vi "ExitNowAllLoops.vi"(8 "error in (no error)":errorcluster, 11 "MessageQues":T1) -> (0 "error out":errorcluster)   [LabVIEW 2019]
doc: "Send ExitNow message to all loops.\n\n Execute all que operations even if there is an error in.\n\nBolder Software LLC"
uses:
  VXM Main Test App/MultipleMessageQues vxm.ctl
  MessageQue.ctl
  MessageCluster.ctl
  MessageQue.lvlib
panel:
  # "SaveData Ques\nDisplay Que\nDisplayNotifier"
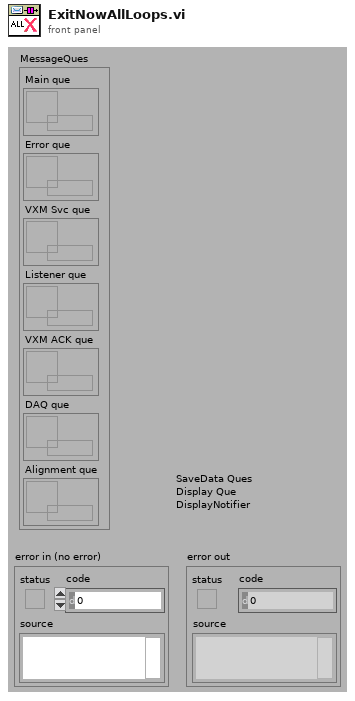
[diagram p1: front panel]
types:
  T1 = typedef "MultipleMessageQues vxm.ctl" = cluster{"Main que":T2, "Error que":T2, "VXM Svc que":T2, "Listener que":T2, "VXM ACK que":T2, "DAQ que":T2, "Alignment que":T2}
  T2 = typedef "MessageQue.lvlib/MessageQue.ctl" = refnum<queue>
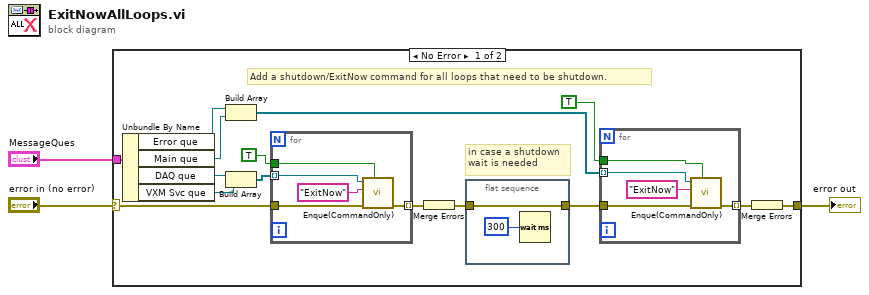
[diagram p0: block diagram]
diagram:
  n1 = case shown="No Error" "error in (no error)" {
    selector: "error in (no error)" -> [w18 w31]
    tunnel: [w11 w31] -> w2
    tunnel: "MessageQues" -> [w15 _]
    frame No Error {
      # "Add a shutdown/ExitNow command for all loops that need to be shutdown."
      # "in case a shutdown\nwait is needed"
      n2 = Unbundle By Name(w15) -> ("Error que"=w6:T2, "Main que"=w5:T2, "DAQ que"=w13:T2, "VXM Svc que"=w4:T2)
      n3 = Build Array(w6, w5) -> (w9:T2[])
      n4 = Build Array(w13, w4) -> (w14:T2[])
      n5 = for {
        tunnel: w18 -> [w30]
        tunnel: TRUE ("at front (F)") -> [w26]
        tunnel: [w29] -> w16 mode=indexing
        tunnel: w14 -> [w27] mode=indexing
        n6 = call "Enque(CommandOnly).vi"("at front (F)"=w26, "error in"=w30, "Message Command"="ExitNow" ("Command"), "Message que"=w27) -> ("error out"=w29:errorcluster)  [unwired: 6 in, 1 out]
      }
      n7 = Merge Errors(w16) -> (w8:errorcluster)
      n8 = flat-sequence {
        tunnel: [w19] -> w7
        tunnel: w8 -> [w19]
        frame #0 {
          n9 = Wait (ms)(milliseconds to wait=u32 300) -> ()  [unwired: 1 out]
        }
      }
      n10 = for {
        tunnel: w7 -> [w24]
        tunnel: TRUE ("at front (F)") -> [w22]
        tunnel: [w23] -> w12 mode=indexing
        tunnel: w9 -> [w21] mode=indexing
        n11 = call "Enque(CommandOnly).vi"("at front (F)"=w22, "error in"=w24, "Message Command"="ExitNow" ("Command"), "Message que"=w21) -> ("error out"=w23:errorcluster)  [unwired: 6 in, 1 out]
      }
      n12 = Merge Errors(w12) -> (w11:errorcluster)
    }
    frame Error {
    }
  }
  "error out" <- w2
